vi "Config Core.vi"(8 "Error In":errorcluster, 10 "ConfigB In":refnum<class "ConfigB.lvclass">, 11 "Hardware In":refnum<class "IRef.lvclass">) -> (0 "Error Out":errorcluster, 2 "ConfigB Out":refnum<class "ConfigB.lvclass">, 3 "Hardware Out":refnum<class "IRef.lvclass">)   [LabVIEW 2020, in "ConfigB.lvclass"]
uses:
  ConfigB.lvclass
  IReference/IRef.lvclass
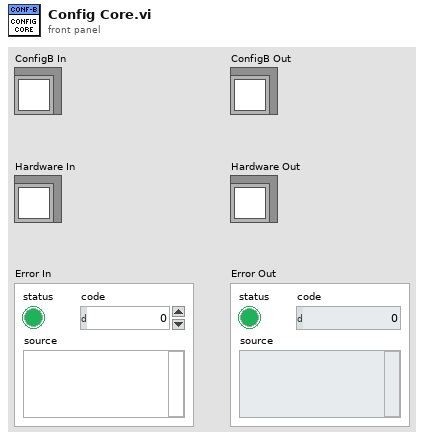
[diagram p1: front panel]
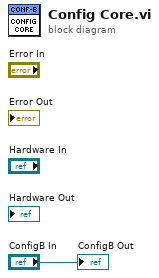
[diagram p0: block diagram]
diagram:
  "ConfigB Out" <- "ConfigB In"
